vi "CCDSingleShotLV7.vi"(4 "The Reference Data In":dbl[](array[numeric]), 5 "Ref Operation In":u8, 6 "error in":errorcluster, 9 "File Info in":T6={"FilePath"=path "", "Field (T)"=0.0, "Temperature (K)"=0.0, "X-Axis"=enum."Point", "Center nm"=0.0, "Current Grating Density"=enum."150", "CCD Parameters"={"Exposure Time (s)"=0.2, "Offset"=0.0, "BkgrdCrct"=FALSE, "Shutter"=FALSE, "Mode"=enum."Regular", "Repetition"=4, "dt or s"=0.0}, "Operation Mode"=enum."Standby", "Exp Index"=0, "Index_repetition"=0, "Index"=0, "Current Detector"=enum."CCD-1024x256"} {"CCD Parameters"."dt or s" format="%#.6f"; "CCD Parameters"."Repetition" min=1; "CCD Parameters"."Offset" format="%#.2f"; "CCD Parameters"."Exposure Time (s)" min=0.02 max=6000.0 format="%#.2f"; "Center nm" format="%.2f"; "Temperature (K)" format="%.2f"; "Field (T)" format="%.2f"}) -> (0 "Error Out":errorcluster, 3 "File Info out":T6={"FilePath"=path "", "Field (T)"=0.0, "Temperature (K)"=0.0, "X-Axis"=enum."Point", "Center nm"=0.0, "Current Grating Density"=enum."150", "CCD Parameters"={"Exposure Time (s)"=0.2, "Offset"=0.0, "BkgrdCrct"=FALSE, "Shutter"=FALSE, "Mode"=enum."Regular", "Repetition"=4, "dt or s"=0.0}, "Operation Mode"=enum."Standby", "Exp Index"=0, "Index_repetition"=0, "Index"=0, "Current Detector"=enum."CCD-1024x256"} {"CCD Parameters"."dt or s" format="%#.6f"; "CCD Parameters"."Repetition" min=1; "CCD Parameters"."Offset" format="%#.2f"; "CCD Parameters"."Exposure Time (s)" min=0.02 max=6000.0 format="%#.2f"; "Center nm" format="%.2f"; "Temperature (K)" format="%.2f"; "Field (T)" format="%.2f"})   [LabVIEW 2021]
uses:
  Globals and TypeDefs/Type Definitions.llb/Wavelength Unit.ctt
  Globals and TypeDefs/Type Definitions.llb/McPherson Grating Density.ctl
  Globals and TypeDefs/Type Definitions.llb/CCDParameter.ctt
  Globals and TypeDefs/Type Definitions.llb/OperationMode.ctt
  Globals and TypeDefs/Type Definitions.llb/ListOfDetectors.ctt
  Globals and TypeDefs/3wayStatus.ctl
  Globals and TypeDefs/gStatus.vi
panel:
  out "Status":string
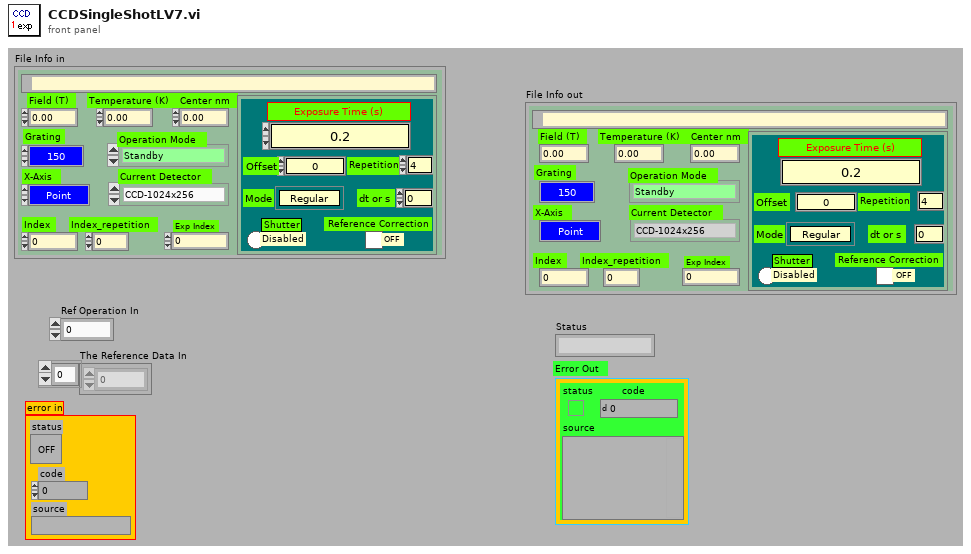
[diagram p1: front panel]
types:
  T1 = typedef "Wavelength Unit.ctt" = enum8{"Point", "nm", "eV", "meV", "cm_1"}
  T2 = typedef "McPherson Grating Density.ctl" = enum8{"150", "300", "600", "1200", "1800"}
  T3 = typedef "CCDParameter.ctt" = cluster{"Exposure Time (s)":dbl, "Offset":dbl, "BkgrdCrct":bool, "Shutter":bool, "Mode":enum8{"Regular", "OverExp Cor", "SpikeRemove", "ForCalibration"}, "Repetition":u16, "dt or s":dbl}
  T4 = typedef "OperationMode.ctt" = enum16{"Standby", "CCD Single Shot", "CCD Sequence Shots", "CCD Custom Shots", "CCD Reference Shot", "Step Scanning ", "Time Scanning", "NML Data Acquisition"}
  T5 = typedef "ListOfDetectors.ctt" = enum8{"CCD-1024x256", "InGaAs PDA-1024x1", "CCD-1340x400", "Ge Single Channel", "Si Single Channel", "PMT Single Channel"}
  T6 = cluster{"FilePath":path, "Field (T)":dbl, "Temperature (K)":dbl, "X-Axis":T1, "Center nm":dbl, "Current Grating Density":T2, "CCD Parameters":T3, "Operation Mode":T4, "Exp Index":u32, "Index_repetition":u16, "Index":u16, "Current Detector":T5}
  T7 = typedef "FileInfoParameter.ctt" = cluster{"FilePath":path, "Field (T)":dbl, "Temperature (K)":dbl, "X-Axis":T1, "Center nm":dbl, "Current Grating Density":T2, "CCD Parameters":T3, "Operation Mode":T4, "Exp Index":u32, "Index_repetition":u16, "Index":u16, "Current Detector":T5}
  T8 = typedef "3wayStatus.ctl" = u8
  T9 = typedef "3 way Status.ctl" = u8
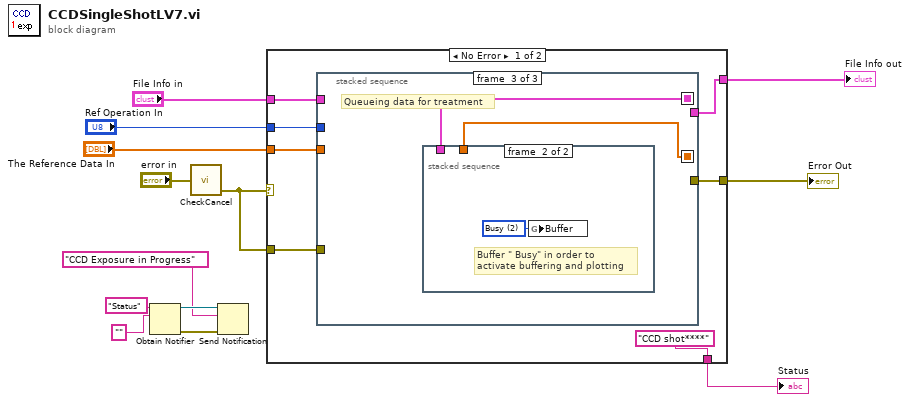
[diagram p0: block diagram]
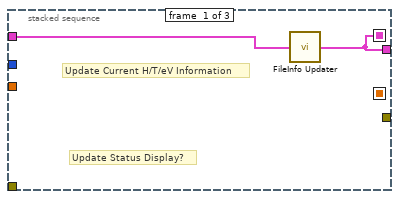
[diagram p2: hidden frame]
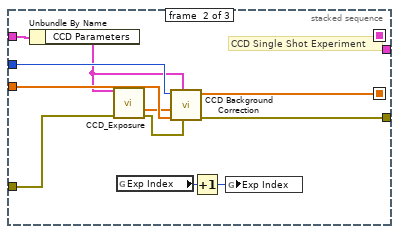
[diagram p3: hidden frame]
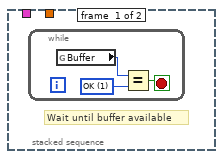
[diagram p4: hidden frame]
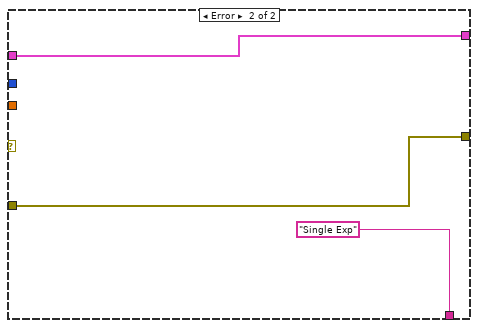
[diagram p5: hidden frame]
diagram:
  n1 = Obtain Notifier(name (unnamed)="Status", notification data type="" ("Status")) -> (notifier out=w3:refnum<notifier>, error out=w2:errorcluster)  [unwired: 2 in, 1 out]
  n2 = call "CheckCancel.vi"("error in (no error)"="error in") -> ("error out"=w6:errorcluster)  [unwired: 1 in, 1 out]
  n3 = Send Notification(notification="CCD Exposure in Progress", notifier=w3, error in (no error)=w2) -> ()  [unwired: 2 out]
  n4 = case shown="No Error" w6 {
    tunnel: "File Info in" -> [w18 w42]
    tunnel: [w17 w42] -> w10
    tunnel: "The Reference Data In" -> [w20 _]
    tunnel: "Ref Operation In" -> [w19 _]
    tunnel: ["CCD shot****" ("Status") "Single Exp" ("Status")] -> w13
    tunnel: w6 -> [w15 w40]
    tunnel: [w14 w40] -> w8
    frame No Error {
      n5 = stacked-sequence {
        seq-local: [w21 _ _] -> [_ _ w35]
        seq-local: [_ w29 _] -> [_ _ w34]
        tunnel: w20 -> [_ w33 _]
        tunnel: w19 -> [_ w32 _]
        tunnel: w18 -> [w22 w31 _]
        tunnel: [w21 _ _] -> w17
        tunnel: w15 -> [_ w24 _]
        tunnel: [_ w23 _] -> w14
        frame #0 {
          # "Update Status Display?"
          # "Update Current H/T/eV Information"
          n6 = call "FileInfo Updater.vi"("File Info"=w22) -> ("File Info output"=w21:T7)
        }
        frame #1 {
          # "CCD Single Shot Experiment"
          n7 = Unbundle By Name(w31) -> ("CCD Parameters"=w30:T3)
          n8 = call "CCD_Exposure.vi"("CCD Parameters"=w30, "error in"=w24) -> ("The Data"=w27:dbl[], "Error Out"=w28:errorcluster)  [unwired: 8 in, 4 out]
          n9 = global read "gStatus.vi" "Exp Index"() -> (w26:u32)
          n10 = call "CCD Background Correction.vi"("error in"=w28, "CCD Parameters"=w30, "The Reference Data In"=w33, "The Signal Data In"=w27, "Operation Mode"=w32) -> ("Error Out"=w23:errorcluster, "The Signal Data Out"=w29:dbl[])  [unwired: 1 in, 2 out]
          n11 = Increment(x=w26) -> (x+1=w25:u32)
          n12 = global write "gStatus.vi" "Exp Index"(w25) -> ()
        }
        frame #2 {
          # "Queueing data for treatment"
          n13 = stacked-sequence {
            tunnel: w34 -> [_ _]
            tunnel: w35 -> [_ _]
            frame #0 {
              # "Wait until buffer available"
              n14 = while {
                stop <- w37 stop-if-true
                w38 = T8 1 items=["N.A.", "OK", "Busy", "Done"] ("y")
                n15 = global read "gStatus.vi" "Buffer"() -> (w36:T9)
                n16 = Equal?(x=w36, y=w38) -> (x = y?=w37:bool)
              }
            }
            frame #1 {
              w39 = T8 2 items=["N.A.", "OK", "Busy", "Done"] ("Buffer")
              # "Buffer \" Busy\" in order to \nactivate buffering and plotting"
              n17 = global write "gStatus.vi" "Buffer"(w39) -> ()
            }
          }
        }
      }
    }
    frame Error {
    }
  }
  "Status" <- w13
  "File Info out" <- w10
  "Error Out" <- w8
